vi "mandibula.vi"() -> ()   [LabVIEW 2025]
uses:
  <vilib>/Instr/_visa.llb/VISA Configure Serial Port (Instr).vi
panel:
  in  "Angulo da Mandibula":dbl(knob) scale=0.0..45.0
  out "2D Picture":picture
  in  "stop":bool
  in  "VISA resource name":refnum<visa-resource-name>
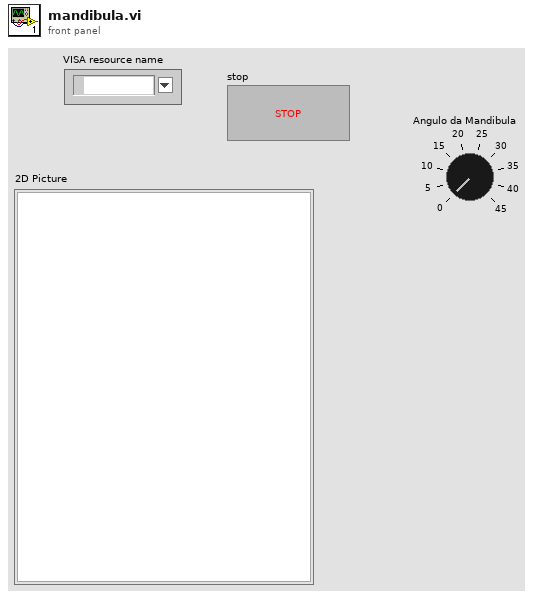
[diagram p1: front panel]
types:
  T1 = typedef "imagedata.ctl" = cluster{"image type":i32, "image depth":i32, "image":u8[], "mask":u8[], "colors":u32[], "Rectangle":cluster{"left":i16, "top":i16, "right":i16, "bottom":i16}}
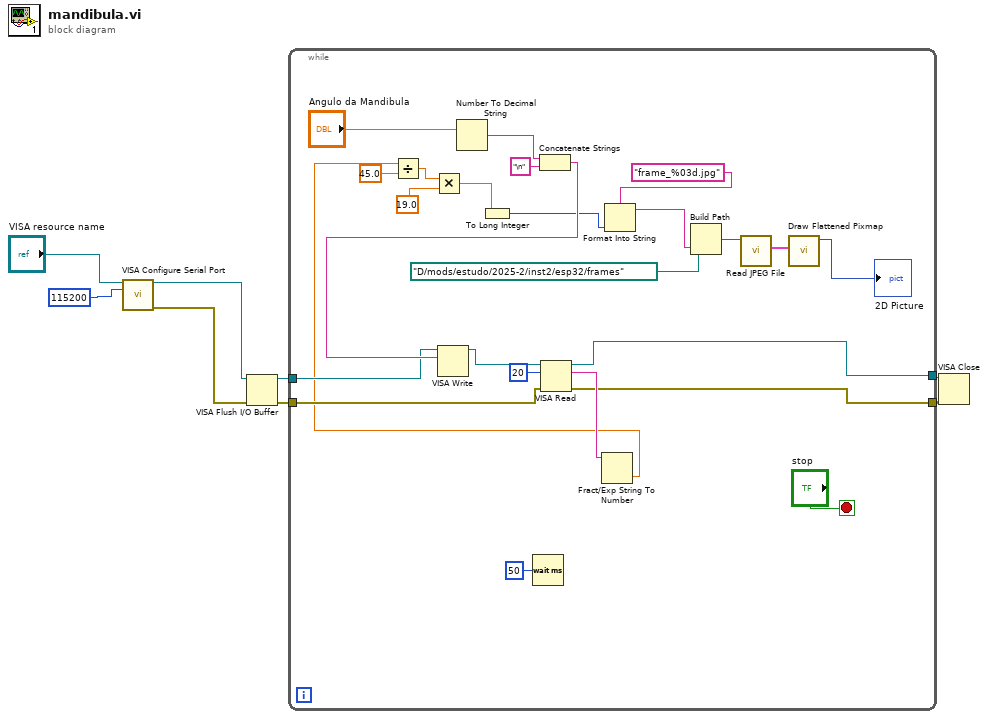
[diagram p0: block diagram]
diagram:
  n1 = call-poly "VISA Configure Serial Port"("VISA resource name"="VISA resource name", "baud rate (9600)"=u32 115200) -> ("VISA resource name out"=w8:refnum<visa-resource-name>, "error out"=w7:errorcluster)  [unwired: 12 in]
  n2 = VISA Flush I/O Buffer(VISA resource name=w8, error in (no error)=w7) -> (VISA resource name out=w6:refnum<visa-resource-name>, error out=w5:errorcluster)  [unwired: 1 in]
  n3 = while {
    tunnel: w6 -> [w26]
    tunnel: w5 -> [w25]
    tunnel: [w24] -> w4
    tunnel: [w23] -> w3
    stop <- "stop" stop-if-true
    n4 = Number To Decimal String(number="Angulo da Mandibula") -> (decimal integer string=w32:string)  [unwired: 1 in]
    n5 = Wait (ms)(milliseconds to wait=u32 50) -> ()  [unwired: 1 out]
    n6 = Concatenate Strings "Concatenate Strings"(w32, "\n" ("string")) -> (w31:string)
    n7 = VISA Write(VISA resource name=w26, write buffer=w31) -> (VISA resource name out=w30:refnum<visa-resource-name>)  [unwired: 1 in, 2 out]
    n8 = VISA Read(VISA resource name=w30, byte count=u32 20, error in (no error)=w25) -> (VISA resource name out=w23:refnum<visa-resource-name>, read buffer=w29:string, error out=w24:errorcluster)  [unwired: 1 out]
    n9 = Fract/Exp String To Number(string=w29) -> (number=w13:dbl)  [unwired: 3 in, 1 out]
    n10 = Divide(x=w13, y=45.0) -> (x/y=w20:dbl)
    n11 = Multiply(x=w20, y=19.0) -> (x*y=w18:dbl)
    n12 = To Long Integer(number=w18) -> (32bit integer=w10:i32)
    n13 = Format Into String(format string="frame_%03d.jpg", w10) -> (resulting string=w11:string)  [unwired: 2 in, 1 out]
    n14 = Build Path(base path=path "D:/mods/estudo/2025-2/inst2/esp32/frames", name or relative path=w11) -> (appended path=w16:path)
    n15 = call <vilib>:"Read JPEG File.vi"("path to JPEG file"=w16) -> ("image data"=w15:T1)  [unwired: 8 in, 2 out]
    n16 = call <vilib>:"Draw Flattened Pixmap.vi"("image data"=w15) -> ("new picture"=→"2D Picture":picture)  [unwired: 8 in]
  }
  n17 = VISA Close(VISA resource name=w3, error in (no error)=w4) -> ()  [unwired: 1 out]
